vi "LabvolutionSubmoduleCheck_Provider_LoadComplete.vi"(11 "reference":refnum<vi>) -> ()   [LabVIEW 2018]
panel:
  out "error out":errorcluster
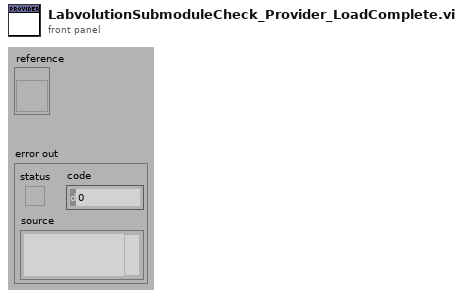
[diagram p1: front panel]
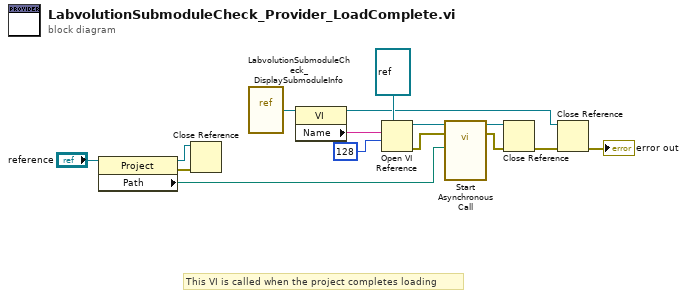
[diagram p0: block diagram]
diagram:
  # "This VI is called when the project completes loading"
  n1 = property class="Project"(reference="reference") -> (reference out=w4:refnum<vi>, error out=w5:errorcluster, "Path"=w6:path)  [unwired: 1 in]
  n2 = Close Reference(reference=w4, error in (no error)=w5) -> ()  [unwired: 1 out]
  n3 = vi-ref "LabvolutionSubmoduleCheck_DisplaySubmoduleInfo.vi"() -> (w14:refnum<vi>)
  n4 = property class="VI"(reference=w14) -> (reference out=w2:refnum<vi>, "Name"=w13:string)  [unwired: 1 in, 1 out]
  n5 = Open VI Reference(type specifier VI Refnum (for type only)=refnum<vi> refnum, vi path=w13, options=128) -> (vi reference=w10:refnum<vi>, error out=w9:errorcluster)  [unwired: 3 in]
  n6 = call-by-ref "Start Asynchronous Call"(reference=w10, error in=w9, "Project Path"=w6) -> (reference out=w8:refnum<vi>, error out=w7:errorcluster)  [unwired: 11 in]
  n7 = Close Reference(reference=w8, error in (no error)=w7) -> (error out=w3:errorcluster)
  n8 = Close Reference(reference=w2, error in (no error)=w3) -> (error out=→"error out":errorcluster)
